vi "ArmController.vi"(2 "Button":bool, 3 "EncoderValues":i32) -> ()   [LabVIEW 2018]
uses:
  Global Variables/ArmLower.vi
  Global Variables/ArmExtend.vi
  Global Variables/ArmWithdraw.vi
  Global Variables/ArmUp.vi
panel:
  in  "EncoderValues 2":i32
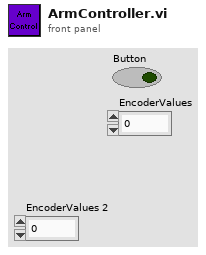
[diagram p1: front panel]
types:
  T1 = typedef "WPI_MotorControlDeviceRef.ctl" = cluster{"DeviceStatus":errorcluster, "Type":T2, "PWM":cluster{"PWM Channel":T3, "DeadBand":T4}, "CAN":cluster{"Device Number":u8, "SetOutput VI Ref":variant, "GetOutput VI Ref":variant, "Enable VI Ref":variant, "Disable VI Ref":variant, "Data":variant}, "Invert":bool, "DIO PWM":cluster{"PWM \"Enable\" Channel":T3, "DIOChannel":T5, "PWM Rate":dbl}}
  T2 = typedef "WPI_MotorControlType.ctl" = enum16{"PWM", "CAN", "DIO PWM"}
  T3 = typedef "FPGA_DIOPWMChannel.ctl" = enum8{"PWM 0", "PWM 1", "PWM 2", "PWM 3", "PWM 4", "PWM 5", "PWM 6", "PWM 7", "PWM 8", "PWM 9", "PWM MXP 0", "PWM MXP 1", "PWM MXP 2", "PWM MXP 3", "PWM MXP 4", "PWM MXP 5", "PWM MXP 6", "PWM MXP 7", "PWM MXP 8", "PWM MXP 9", "Invalid"}
  T4 = typedef "WPI_PWMDeadband.ctl" = cluster{"Name":string, "maxPositivePwm":i32, "minPositivePwm":i32, "centerPwm":i32, "maxNegativePwm":i32, "minNegativePwm":i32, "angularRange":u16}
  T5 = typedef "FPGA_DIOChannel.ctl" = enum8{"DIO 0", "DIO 1", "DIO 2", "DIO 3", "DIO 4", "DIO 5", "DIO 6", "DIO 7", "DIO 8", "DIO 9", "DIO MXP 0", "DIO MXP 1", "DIO MXP 2", "DIO MXP 3", "DIO MXP 4", "DIO MXP 5", "DIO MXP 6", "DIO MXP 7", "DIO MXP 8", "DIO MXP 9", "DIO MXP 10", "DIO MXP 11", "DIO MXP 12", "DIO MXP 13", "DIO MXP 14", "DIO MXP 15", "SPI Port CS1", "SPI Port CS2", "SPI Port CS3", "SPI Port MISO", "SPI Port MOSI", "Invalid"}
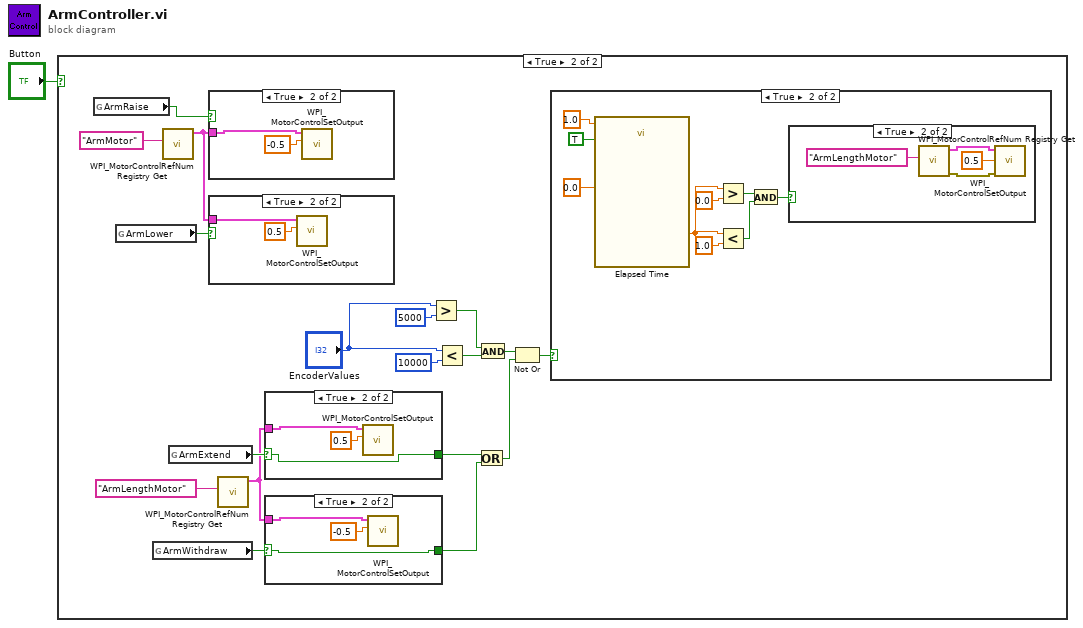
[diagram p0: block diagram]
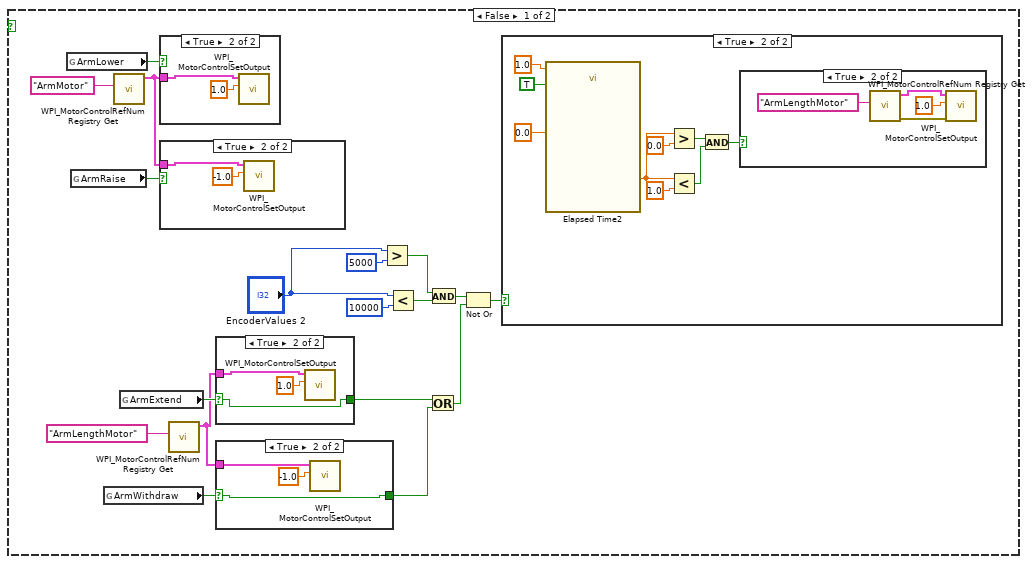
[diagram p2: hidden frame]
diagram:
  n1 = case shown="True" "Button" {
    frame False {
      n2 = global read "ArmLower.vi" "ArmLower"() -> (w19:bool)
      n3 = global read "ArmUp.vi" "ArmRaise"() -> (w2:bool)
      n4 = global read "ArmWithdraw.vi" "ArmWithdraw"() -> (w17:bool)
      n5 = call <vilib>:"WPI_MotorControlRefNum Registry Get.vi"("refnum name"="ArmMotor") -> ("MotorControlDevRef"=w15:T1)  [unwired: 9 in, 1 out]
      n6 = global read "ArmExtend.vi" "ArmExtend"() -> (w18:bool)
      n7 = case shown="True" w19 {
        tunnel: w15 -> [_ w42]
        frame False {
        }
        frame True {
          n8 = call <vilib>:"WPI_MotorControlSetOutput.vi"("Output"=1.0, "MotorControlDevRef"=w42) -> ()  [unwired: 7 in, 3 out]
        }
      }
      n9 = case shown="True" w2 {
        tunnel: w15 -> [_ w44]
        frame False {
        }
        frame True {
          n10 = call <vilib>:"WPI_MotorControlSetOutput.vi"("Output"=-1.0, "MotorControlDevRef"=w44) -> ()  [unwired: 7 in, 3 out]
        }
      }
      n11 = call <vilib>:"WPI_MotorControlRefNum Registry Get.vi"("refnum name"="ArmLengthMotor") -> ("MotorControlDevRef"=w13:T1)  [unwired: 9 in, 1 out]
      n12 = case shown="True" w18 {
        selector: w18 -> [w37 w38]
        tunnel: w13 -> [_ w40]
        tunnel: [w37 w38] -> w7
        frame False {
        }
        frame True {
          n13 = call <vilib>:"WPI_MotorControlSetOutput.vi"("Output"=1.0, "MotorControlDevRef"=w40) -> ()  [unwired: 7 in, 3 out]
        }
      }
      n14 = case shown="True" w17 {
        selector: w17 -> [w33 w34]
        tunnel: w13 -> [_ w36]
        tunnel: [w33 w34] -> w6
        frame False {
        }
        frame True {
          n15 = call <vilib>:"WPI_MotorControlSetOutput.vi"("Output"=-1.0, "MotorControlDevRef"=w36) -> ()  [unwired: 7 in, 3 out]
        }
      }
      n16 = Greater?(x="EncoderValues 2", y=5000) -> (0:w12:bool)
      n17 = Less?(x="EncoderValues 2", y=10000) -> (x < y?=w11:bool)
      n18 = Or(x=w7, y=w6) -> (x .or. y?=w4:bool)
      n19 = And(x=w12, y=w11) -> (x .and. y?=w5:bool)
      n20 = Not Or(1:w4, 2:w5) -> (0:w3:bool)
      n21 = case shown="True" w3 {
        frame False {
        }
        frame True {
          n22 = call "Elapsed Time2"("Time Target (s)"=1.0, "Reset"=TRUE ("Auto Reset"), "Set Start Time (s)"=0.0) -> ("Elapsed Time (s)"=w24:dbl)  [unwired: 9 in, 7 out]
          n23 = Greater?(x=w24, y=0.0) -> (0:w27:bool)
          n24 = Less?(x=w24, y=1.0) -> (x < y?=w28:bool)
          n25 = And(x=w27, y=w28) -> (x .and. y?=w26:bool)
          n26 = case shown="True" w26 {
            frame False {
            }
            frame True {
              n27 = call <vilib>:"WPI_MotorControlRefNum Registry Get.vi"("refnum name"="ArmLengthMotor") -> ("error out"=w31:errorcluster, "MotorControlDevRef"=w32:T1)  [unwired: 9 in]
              n28 = call <vilib>:"WPI_MotorControlSetOutput.vi"("error in (no error)"=w31, "Output"=1.0, "MotorControlDevRef"=w32) -> ()  [unwired: 6 in, 3 out]
            }
          }
        }
      }
    }
    frame True {
      n29 = global read "ArmUp.vi" "ArmRaise"() -> (w45:bool)
      n30 = global read "ArmLower.vi" "ArmLower"() -> (w62:bool)
      n31 = global read "ArmWithdraw.vi" "ArmWithdraw"() -> (w60:bool)
      n32 = call <vilib>:"WPI_MotorControlRefNum Registry Get.vi"("refnum name"="ArmMotor") -> ("MotorControlDevRef"=w58:T1)  [unwired: 9 in, 1 out]
      n33 = global read "ArmExtend.vi" "ArmExtend"() -> (w61:bool)
      n34 = case shown="True" w45 {
        tunnel: w58 -> [_ w87]
        frame False {
        }
        frame True {
          n35 = call <vilib>:"WPI_MotorControlSetOutput.vi"("Output"=-0.5, "MotorControlDevRef"=w87) -> ()  [unwired: 7 in, 3 out]
        }
      }
      n36 = case shown="True" w62 {
        tunnel: w58 -> [_ w85]
        frame False {
        }
        frame True {
          n37 = call <vilib>:"WPI_MotorControlSetOutput.vi"("Output"=0.5, "MotorControlDevRef"=w85) -> ()  [unwired: 7 in, 3 out]
        }
      }
      n38 = call <vilib>:"WPI_MotorControlRefNum Registry Get.vi"("refnum name"="ArmLengthMotor") -> ("MotorControlDevRef"=w56:T1)  [unwired: 9 in, 1 out]
      n39 = case shown="True" w61 {
        selector: w61 -> [w80 w81]
        tunnel: w56 -> [_ w83]
        tunnel: [w80 w81] -> w50
        frame False {
        }
        frame True {
          n40 = call <vilib>:"WPI_MotorControlSetOutput.vi"("Output"=0.5, "MotorControlDevRef"=w83) -> ()  [unwired: 7 in, 3 out]
        }
      }
      n41 = case shown="True" w60 {
        selector: w60 -> [w76 w77]
        tunnel: w56 -> [_ w79]
        tunnel: [w76 w77] -> w49
        frame False {
        }
        frame True {
          n42 = call <vilib>:"WPI_MotorControlSetOutput.vi"("Output"=-0.5, "MotorControlDevRef"=w79) -> ()  [unwired: 7 in, 3 out]
        }
      }
      n43 = Greater?(x="EncoderValues", y=5000) -> (0:w55:bool)
      n44 = Less?(x="EncoderValues", y=10000) -> (x < y?=w54:bool)
      n45 = Or(x=w50, y=w49) -> (x .or. y?=w47:bool)
      n46 = And(x=w55, y=w54) -> (x .and. y?=w48:bool)
      n47 = Not Or(1:w47, 2:w48) -> (0:w46:bool)
      n48 = case shown="True" w46 {
        frame False {
        }
        frame True {
          n49 = call "Elapsed Time"("Time Target (s)"=1.0, "Reset"=TRUE ("Auto Reset"), "Set Start Time (s)"=0.0) -> ("Elapsed Time (s)"=w67:dbl)  [unwired: 9 in, 7 out]
          n50 = Greater?(x=w67, y=0.0) -> (0:w70:bool)
          n51 = Less?(x=w67, y=1.0) -> (x < y?=w71:bool)
          n52 = And(x=w70, y=w71) -> (x .and. y?=w69:bool)
          n53 = case shown="True" w69 {
            frame False {
            }
            frame True {
              n54 = call <vilib>:"WPI_MotorControlRefNum Registry Get.vi"("refnum name"="ArmLengthMotor") -> ("error out"=w74:errorcluster, "MotorControlDevRef"=w75:T1)  [unwired: 9 in]
              n55 = call <vilib>:"WPI_MotorControlSetOutput.vi"("error in (no error)"=w74, "Output"=0.5, "MotorControlDevRef"=w75) -> ()  [unwired: 6 in, 3 out]
            }
          }
        }
      }
    }
  }
